vi "getPositionsAndVoltages.vi"(0 "connection ID":refnum<k5>, 5 "error":errorcluster) -> (12 "val2":i32, 13 "val3":i32, 14 "connection ID out":refnum<k5>, 15 "pos1":dbl, 16 "pos2":dbl, 17 "pos3":dbl, 18 "val1":i32, 19 "error out":errorcluster)   [LabVIEW 2016, in "amc_api.lvlib"]
doc: "Simultaneously get 3 axes positions as well as the DC offset\n position-value is -2147483648 nm, if sensor is disabled or no positioner is connected."
uses:
  amc_api.lvlib
panel:
  out "jsonRespIn":string
  out "JSON-response":string="{\"jsonrpc\":\"2.0\",\"method\":\"\",\"params\":[5,1.245,true,\"name\"],\"id\":\"1\"}"
  out "JSON request":string
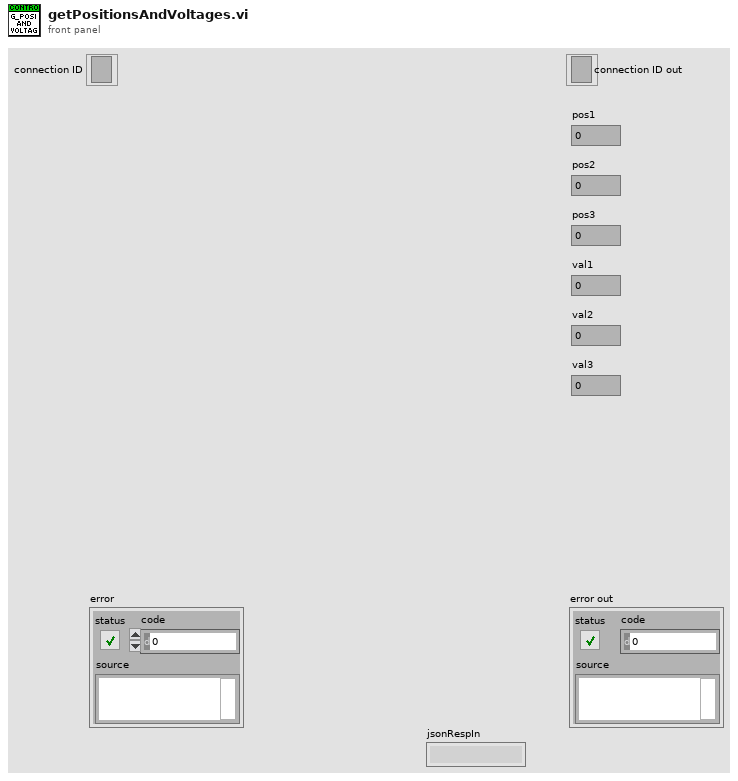
[diagram p1: front panel]
types:
  T1 = cluster{"jsonrpc":string, "method":string, "params":string[], "id":string, "api":i32, "pid":string}
  T2 = enum16{"Standard", "Buffered", "CRLF", "Immediate"}
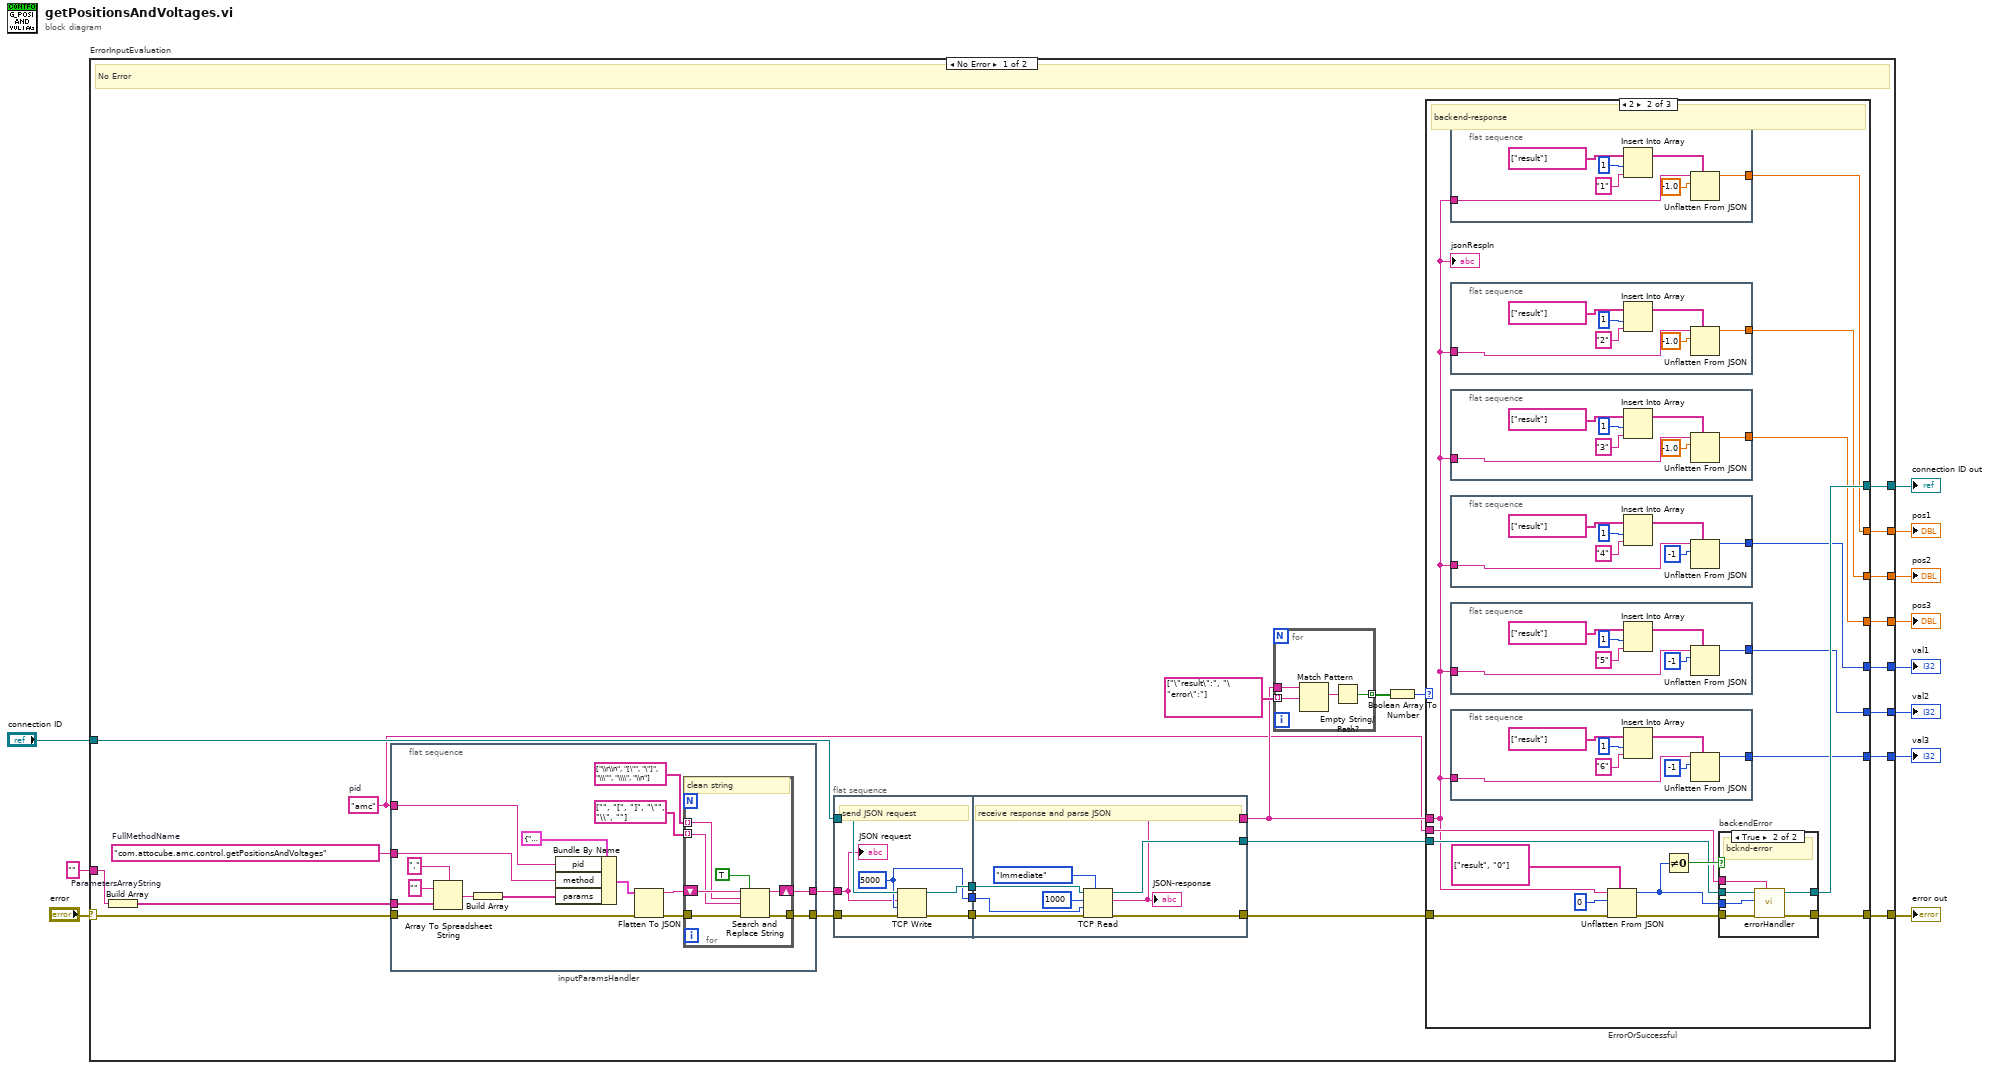
[diagram p0: block diagram]
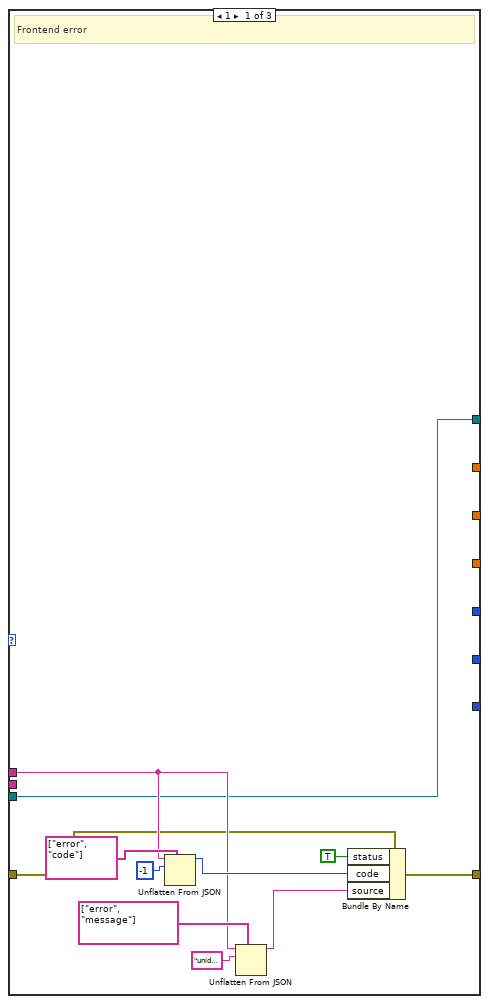
[diagram p2: hidden frame]
diagram:
  n1 = case "ErrorInputEvaluation" shown="No Error" "error" {
    selector: "error" -> [w29 w158]
    tunnel: "connection ID" -> [w33 w159]
    tunnel: [w20 w158] -> w10
    tunnel: [w21 w159] -> w9
    tunnel: "" -> [w18 _]
    tunnel: [w17 _] -> w6
    tunnel: [w16 _] -> w5
    tunnel: [w15 _] -> w4
    tunnel: [w14 _] -> w3
    tunnel: [w13 _] -> w2
    tunnel: [w12 _] -> w1
    frame No Error {
      w19 = "amc"  # pid
      w30 = "com.attocube.amc.control.getPositionsAndVoltages"  # FullMethodName
      # "No Error"
      n2 = Build Array "ParametersArrayString"(w18) -> (w28:string[])
      n3 = flat-sequence "inputParamsHandler" {
        tunnel: [w122] -> w27
        tunnel: w28 -> [w128]
        tunnel: w29 -> [w127]
        tunnel: [w124] -> w26
        tunnel: w30 -> [w118]
        tunnel: w19 -> [w117]
        frame #0 {
          n4 = Array To Spreadsheet String(delimiter (Tab)=",", array=w128, 3:"" ("format string")) -> (spreadsheet string=w130:string)
          n5 = Build Array "Build Array"(w130) -> (w119:string[])
          n6 = Bundle By Name(cluster=T1 {"jsonrpc"="2.0", "method"="com.attocube.amc.res.setRESReadOutFreq", "params"=[], "id"="1", "api"=2, "pid"=""} ("Cluster"), "pid"=w117, "method"=w118, "params"=w119) -> (w129:T1)
          n7 = Flatten To JSON(anything=w129, error in (no error)=w127) -> (JSON string=w123:string, 11:w125:errorcluster)  [unwired: 1 in]
          n8 = for {
            tunnel: string[] ["\\r\\n", "[\"", "\"]", "\\\"", "\\\\", "\\n"] ("search string") -> [w136] mode=indexing
            tunnel: string[] ["", "[", "]", "\"", "\\", ""] ("replace string (\"\")") -> [w135] mode=indexing
            shift-right: [w138] -> w122
            shift-left: w123 -> [w137]
            tunnel: w125 -> [w134]
            tunnel: [w133] -> w124
            # "clean string"
            n9 = Search and Replace String(replace all?=TRUE ("replace all? (F)"), input string=w137, search string=w136, replace string=w135, error in=w134) -> (result string=w138:string, error out=w133:errorcluster)  [unwired: 3 in, 2 out]
          }
        }
      }
      n10 = flat-sequence {
        tunnel: w33 -> [w149]
        tunnel: [w147] -> w36
        tunnel: [w148] -> w35
        tunnel: w26 -> [w144]
        tunnel: [w146] -> w34
        tunnel: w27 -> [w145]
        tunnel: [w153] -> w25
        tunnel: w36 -> [w155]
        tunnel: w35 -> [w154]
        tunnel: [w151] -> w24
        tunnel: w34 -> [w152]
        tunnel: [w150] -> w23
        frame #0 {
          w146 = 5000 ("timeout ms (25000)")
          # "send JSON request"
          n11 = TCP Write(connection ID=w149, data in=w145, error in (no error)=w144, 9:w146) -> (connection ID out=w147:refnum<k5>, error out=w148:errorcluster)  [unwired: 1 out]
          "JSON request" <- w145
        }
        frame #1 {
          # "receive response and parse JSON"
          n12 = TCP Read(connection ID=w155, bytes to read=1000, error in (no error)=w154, 7:T2."Immediate" ("mode (standard)"), 9:w152) -> (connection ID out=w153:refnum<k5>, data out=w150:string, error out=w151:errorcluster)
          "JSON-response" <- w150
        }
      }
      n13 = for {
        tunnel: string[] ["\"result\":", "\"error\":"] ("path") -> [w142] mode=indexing
        tunnel: [w140] -> w31 mode=indexing
        tunnel: w23 -> [w143]
        n14 = Match Pattern(string=w143, regular expression=w142) -> (match substring=w141:string)  [unwired: 1 in, 3 out]
        n15 = Empty String/Path?(string/path=w141) -> (empty?=w140:bool)
      }
      n16 = Boolean Array To Number(Boolean array=w31) -> (number=w22:u32)
      n17 = case "ErrorOrSuccessful" shown="2" w22 {
        tunnel: w23 -> [w39 w56 _]
        tunnel: w25 -> [w37 w58 w116]
        tunnel: [w37 w57 w116] -> w21
        tunnel: [w40 w54 w115] -> w20
        tunnel: w24 -> [w38 w55 w115]
        tunnel: w19 -> [_ w59 _]
        tunnel: [_ w53 _] -> w17
        tunnel: [_ w52 _] -> w16
        tunnel: [_ w51 _] -> w15
        tunnel: [_ w50 _] -> w14
        tunnel: [_ w49 _] -> w13
        tunnel: [_ w48 _] -> w12
        frame 1 {
          # "Frontend error"
          n18 = Unflatten From JSON(path=string[] ["error", "code"], JSON string=w39, type and defaults=-1) -> (value=w46:i32)  [unwired: 4 in, 1 out]
          n19 = Unflatten From JSON(path=string[] ["error", "message"], JSON string=w39, type and defaults="unidentified error") -> (value=w47:string)  [unwired: 4 in, 1 out]
          n20 = Bundle By Name(cluster=w38, "status"=TRUE, "code"=w46, "source"=w47) -> (w40:errorcluster)
        }
        frame 2 {
          # "backend-response"
          n21 = flat-sequence "out_double" {
            tunnel: [w100] -> w53
            tunnel: w56 -> [w102]
            frame #0 {
              n22 = Insert Into Array(array=string[] ["result"] ("path"), index=1, new element="1" ("idx")) -> (w104:string[])
              n23 = Unflatten From JSON(path=w104, JSON string=w102, type and defaults=-1.0 ("index")) -> (value=w100:dbl)  [unwired: 4 in, 1 out]
            }
          }
          n24 = flat-sequence "out_double" {
            tunnel: [w93] -> w52
            tunnel: w56 -> [w95]
            frame #0 {
              n25 = Insert Into Array(array=string[] ["result"] ("path"), index=1, new element="2" ("idx")) -> (w97:string[])
              n26 = Unflatten From JSON(path=w97, JSON string=w95, type and defaults=-1.0 ("index")) -> (value=w93:dbl)  [unwired: 4 in, 1 out]
            }
          }
          n27 = flat-sequence "out_double" {
            tunnel: [w86] -> w51
            tunnel: w56 -> [w88]
            frame #0 {
              n28 = Insert Into Array(array=string[] ["result"] ("path"), index=1, new element="3" ("idx")) -> (w90:string[])
              n29 = Unflatten From JSON(path=w90, JSON string=w88, type and defaults=-1.0 ("index")) -> (value=w86:dbl)  [unwired: 4 in, 1 out]
            }
          }
          n30 = flat-sequence "out_integer" {
            tunnel: w56 -> [w81]
            tunnel: [w79] -> w50
            frame #0 {
              n31 = Insert Into Array(array=string[] ["result"] ("path"), index=1, new element="4" ("idx")) -> (w83:string[])
              n32 = Unflatten From JSON(path=w83, JSON string=w81, type and defaults=-1 ("index")) -> (value=w79:i32)  [unwired: 4 in, 1 out]
            }
          }
          n33 = flat-sequence "out_integer" {
            tunnel: w56 -> [w74]
            tunnel: [w72] -> w49
            frame #0 {
              n34 = Insert Into Array(array=string[] ["result"] ("path"), index=1, new element="5" ("idx")) -> (w76:string[])
              n35 = Unflatten From JSON(path=w76, JSON string=w74, type and defaults=-1 ("index")) -> (value=w72:i32)  [unwired: 4 in, 1 out]
            }
          }
          n36 = flat-sequence "out_integer" {
            tunnel: w56 -> [w67]
            tunnel: [w65] -> w48
            frame #0 {
              n37 = Insert Into Array(array=string[] ["result"] ("path"), index=1, new element="6" ("idx")) -> (w69:string[])
              n38 = Unflatten From JSON(path=w69, JSON string=w67, type and defaults=-1 ("index")) -> (value=w65:i32)  [unwired: 4 in, 1 out]
            }
          }
          n39 = Unflatten From JSON(path=string[] ["result", "0"], JSON string=w56, type and defaults=0, error in (no error)=w55) -> (value=w60:i32, error out=w62:errorcluster)  [unwired: 3 in]
          n40 = Not Equal To 0?(x=w60) -> (x != 0?=w61:bool)
          n41 = case "backendError" shown="True" w61 {
            tunnel: w60 -> [_ w114]
            tunnel: w62 -> [w108 w113]
            tunnel: [w107 w112] -> w57
            tunnel: [w108 w111] -> w54
            tunnel: w58 -> [w107 w110]
            tunnel: w59 -> [_ w109]
            frame False {
              # "successful"
            }
            frame True {
              # "bcknd-error"
              n42 = call "errorHandler.vi"("pid"=w109, "error in"=w113, "errNbr"=w114, "connection ID"=w110) -> ("error out 2"=w111:errorcluster, "connection ID out"=w112:refnum<k5>)  [unwired: 6 in]
            }
          }
          "jsonRespIn" <- w56
        }
        frame Default {
          # "NoResponse"
        }
      }
    }
    frame Error {
      # "Error"
    }
  }
  "error out" <- w10
  "connection ID out" <- w9
  "pos1" <- w6
  "pos2" <- w5
  "pos3" <- w4
  "val1" <- w3
  "val2" <- w2
  "val3" <- w1
